vi "20150827 accel+gyro test.vi"() -> ()   [LabVIEW 2013]
uses:
  <vilib>/MakerHub/LINX/Public/Sensors/Accelerometer/MPU60X0/DeviceAddresses.ctl
  <vilib>/MakerHub/LINX/Public/Sensors/Accelerometer/MPU60X0/MPU60X0.lvlib
  <vilib>/MakerHub/LINX/LMH-LINX.lvlib
panel:
  out "Gyro":T1(graph)
  out "Accel":T1(graph)
  in  "Serial Port":refnum<visa-resource-name>="COM10"
  in  "stop":bool
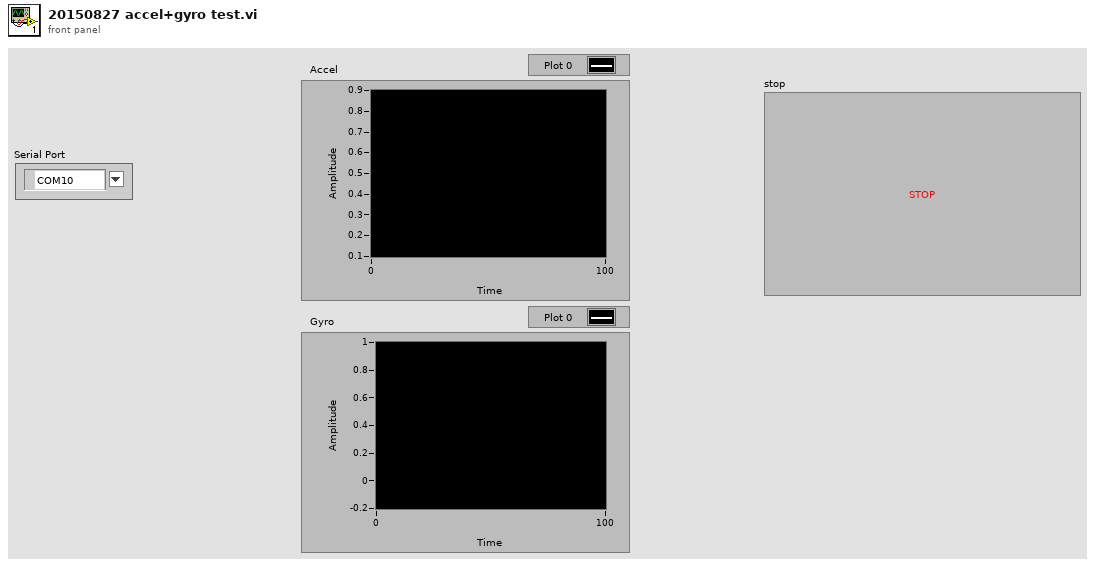
[diagram p1: front panel]
types:
  T1 = cluster{"X Axis":dbl, "Y Axis":dbl, "Z Axis":dbl}
  T2 = typedef "LMH-LINX.lvlib/MPU60X0.lvlib/DeviceAddresses.ctl" = enum16{"0x68", "0x69"}
  T3 = typedef "LMH-LINX.lvlib/LINX Ref.ctl" = cluster{"Platform":T4, "Interface":T5, "LINX Device Config":T6}
  T4 = typedef "LMH-LINX.lvlib/Platform.ctl" = enum16{"LINX", "myRIO"}
  T5 = typedef "LMH-LINX.lvlib/Interface.ctl" = enum16{"Serial", "TCP"}
  T6 = typedef "LMH-LINX.lvlib/Device.lvlib/LINX Device Config.ctl" = cluster{"Interface":T5, "COM Port":refnum<visa-resource-name>, "TCP Configuration":T7, "Device Family":u8, "Device ID":u8, "Device Name":string, "TCP Ref":refnum<k5>, "Channels":T8}
  T7 = typedef "LMH-LINX.lvlib/Device.lvlib/TCP Config.ctl" = cluster{"IP Address":string, "Port":u16}
  T8 = typedef "LMH-LINX.lvlib/Channels.ctl" = cluster{"DI":u8[], "DO":u8[], "AI":u8[], "AO":u8[], "PWM":u8[], "QE":u8[], "UART":u8[], "I2C 2":u8[], "SPI":u8[], "CAN":u8[], "Servo":u8[], "AI Ref (V)":dbl, "AO Ref (V)":dbl, "AO Resolution (Bits)":u8}
  T9 = cluster{"X Axis":i16, "Y Axis":i16, "Z Axis":i16}
  T10 = cluster{"X Axis":i32, "Y Axis":i32, "Z Axis":i32}
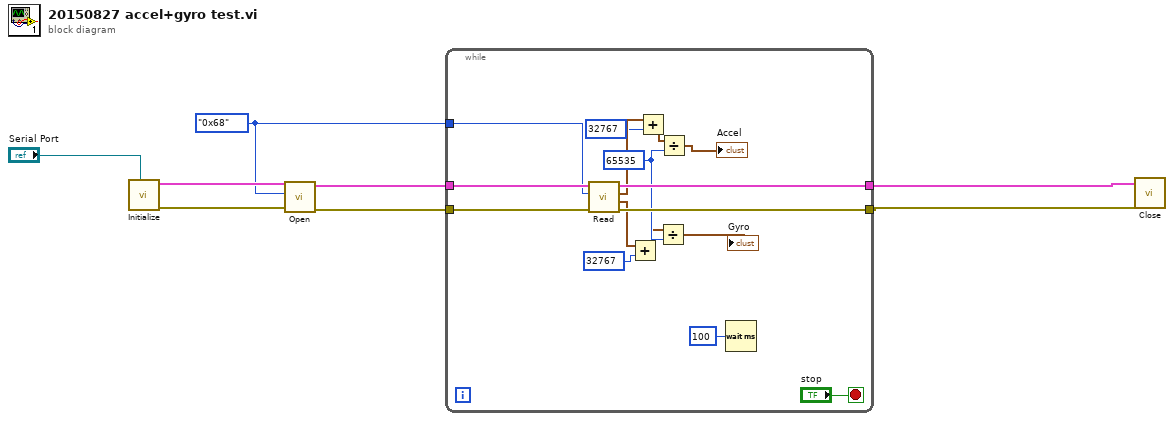
[diagram p0: block diagram]
diagram:
  w3 = DeviceAddresses."0x68" ("Device Address")
  n1 = call <vilib>:"Initialize.vi"("Serial Port"="Serial Port") -> ("Error Out"=w5:errorcluster, "LINX Ref"=w6:T3)  [unwired: 8 in, 1 out]
  n2 = call <vilib>:"Open.vi"("Error In"=w5, "Device Address"=w3, "LINX Resource"=w6) -> ("Error Out"=w7:errorcluster, "LINX Resource"=w8:T3)  [unwired: 7 in]
  n3 = while {
    tunnel: w8 -> [w24]
    tunnel: w7 -> [w23]
    tunnel: [w22] -> w2
    tunnel: [w21] -> w1
    tunnel: w3 -> [w18]
    stop <- "stop" stop-if-true
    w13 = 65535
    n4 = call <vilib>:"Read.vi"("Error In"=w23, "Device Address"=w18, "LINX Resource"=w24) -> ("Error Out"=w21:errorcluster, "Gyro  Data"=w10:T9, "Acceleration Data"=w15:T9, "LINX Resource"=w22:T3)  [unwired: 4 in, 1 out]
    n5 = Add(x=w10, y=32767) -> (x+y=w9:T10)
    n6 = Add(x=w15, y=32767) -> (x+y=w14:T10)
    n7 = Divide(x=w9, y=w13) -> (x/y=→"Gyro":T1)
    n8 = Divide(x=w14, y=w13) -> (x/y=→"Accel":T1)
    n9 = Wait (ms)(milliseconds to wait=u32 100) -> ()  [unwired: 1 out]
  }
  n10 = call <vilib>:"Close.vi"("Error In"=w1, "LINX Resource"=w2) -> ()  [unwired: 8 in, 2 out]
